vi "MEScope_CalStruct_Init.vi"() -> (0 "return type":i32, 8 "error out":errorcluster)   [LabVIEW 2015]
uses:
  ScannerDiagDLL.dll
panel:
  in  "error in (no error)":errorcluster
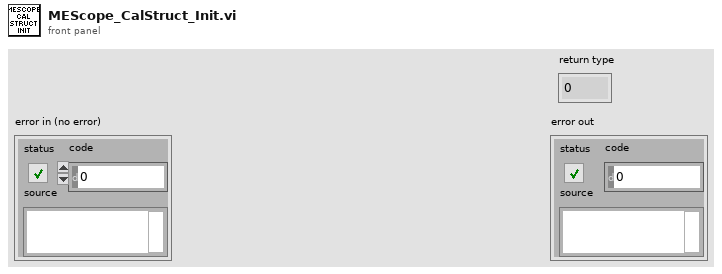
[diagram p1: front panel]
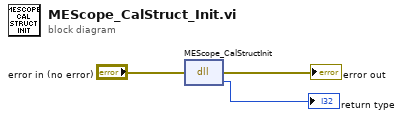
[diagram p0: block diagram]
diagram:
  n1 = dll-call lib="C:/ModisEdge/Scope/Test Sequence/Code Modules/DLL/ScannerDiagDLL.dll" fn="MEScope_CalStructInit"(error in="error in (no error)") -> (error out=→"error out":errorcluster, "return type"=→"return type":i32)  [unwired: 2 in, 1 out]
